vi "Toolkit Error Handling - API VI List Buffer Core.vi"(8 "error in (no error)":errorcluster, 10 "API VI to add (\"\": get list)":string) -> (0 "error out":errorcluster, 2 "API VI List":string[](array[string]))   [LabVIEW 2013]
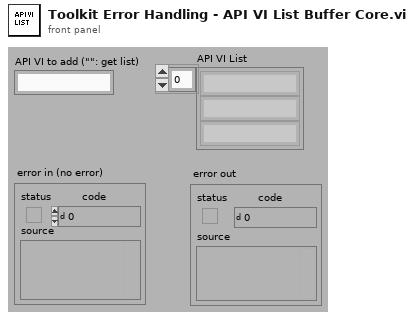
[diagram p1: front panel]
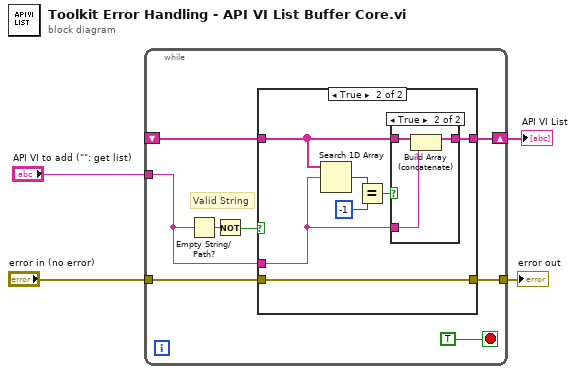
[diagram p0: block diagram]
diagram:
  n1 = while {
    tunnel: "API VI to add (\"\": get list)" -> [w9]
    tunnel: [w8] -> w2
    tunnel: "error in (no error)" -> [w7]
    shift-right: [w5] -> w1
    shift-left: _ -> [w6]
    stop <- TRUE stop-if-true
    # "Valid String"
    n2 = Empty String/Path?(string/path=w9) -> (empty?=w11:bool)
    n3 = Not(x=w11) -> (.not. x?=w10:bool)
    n4 = case shown="True" w10 {
      tunnel: w9 -> [_ w17]
      tunnel: w7 -> [w13 w15]
      tunnel: [w13 w15] -> w8
      tunnel: [w14 w16] -> w5
      tunnel: w6 -> [w14 w18]
      frame False {
      }
      frame True {
        n5 = Search 1D Array(1D array=w18, element=w17) -> (index of element=w21:i32)  [unwired: 1 in]
        n6 = Equal?(x=w21, y=-1) -> (x = y?=w19:bool)
        n7 = case shown="True" w19 {
          tunnel: w18 -> [w22 w25]
          tunnel: w17 -> [_ w24]
          tunnel: [w22 w23] -> w16
          frame False {
          }
          frame True {
            n8 = Build Array (concatenate)(w25, w24) -> (w23:string[])
          }
        }
      }
    }
  }
  "error out" <- w2
  "API VI List" <- w1
